vi "SubVI_ResAcc3.vi"() -> (0 "error out":errorcluster caption="에러 출력", 3 "data":waveform(dbl)[](array[waveform]) caption="데이터")   [LabVIEW 2016]
uses:
  <vilib>/DAQmx/read.llb/DAQmx Read.vi
  <vilib>/DAQmx/read.llb/DAQmx Read (Analog 1D Wfm NChan NSamp).vi
  <vilib>/DAQmx/create/channels.llb/DAQmx Create Channel (TEDS-AI-Voltage-Basic).vi
  <vilib>/DAQmx/create/channels.llb/DAQmx Create Channel (AI-Voltage-Basic).vi
  <vilib>/DAQmx/configure/timing.llb/DAQmx Timing (Sample Clock).vi
  <vilib>/DAQmx/configure/trigger.llb/DAQmx Trigger.vi
  <vilib>/DAQmx/configure/trigger.llb/DAQmx Start Trigger (Digital Edge).vi
  <vilib>/DAQmx/miscellaneous.llb/DAQmx Fill In Error Info.vi
panel:
  out "웨이브폼 그래프":waveform(dbl)[](graph)
  out "task out":refnum<k21> caption="태스크 출력"
  in  "error in":errorcluster caption="에러 입력"
  in  "stop (T)":bool=TRUE caption="정지(T)"
  in  "속도":dbl=100000.0
  in  "샘플 개수":i32=2000
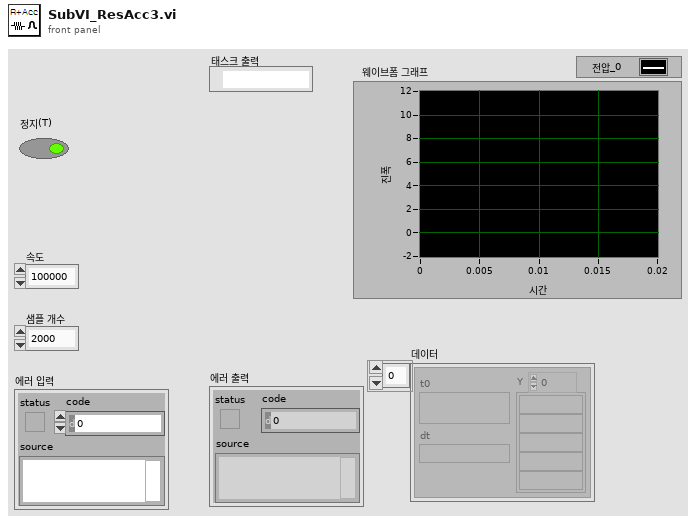
[diagram p1: front panel]
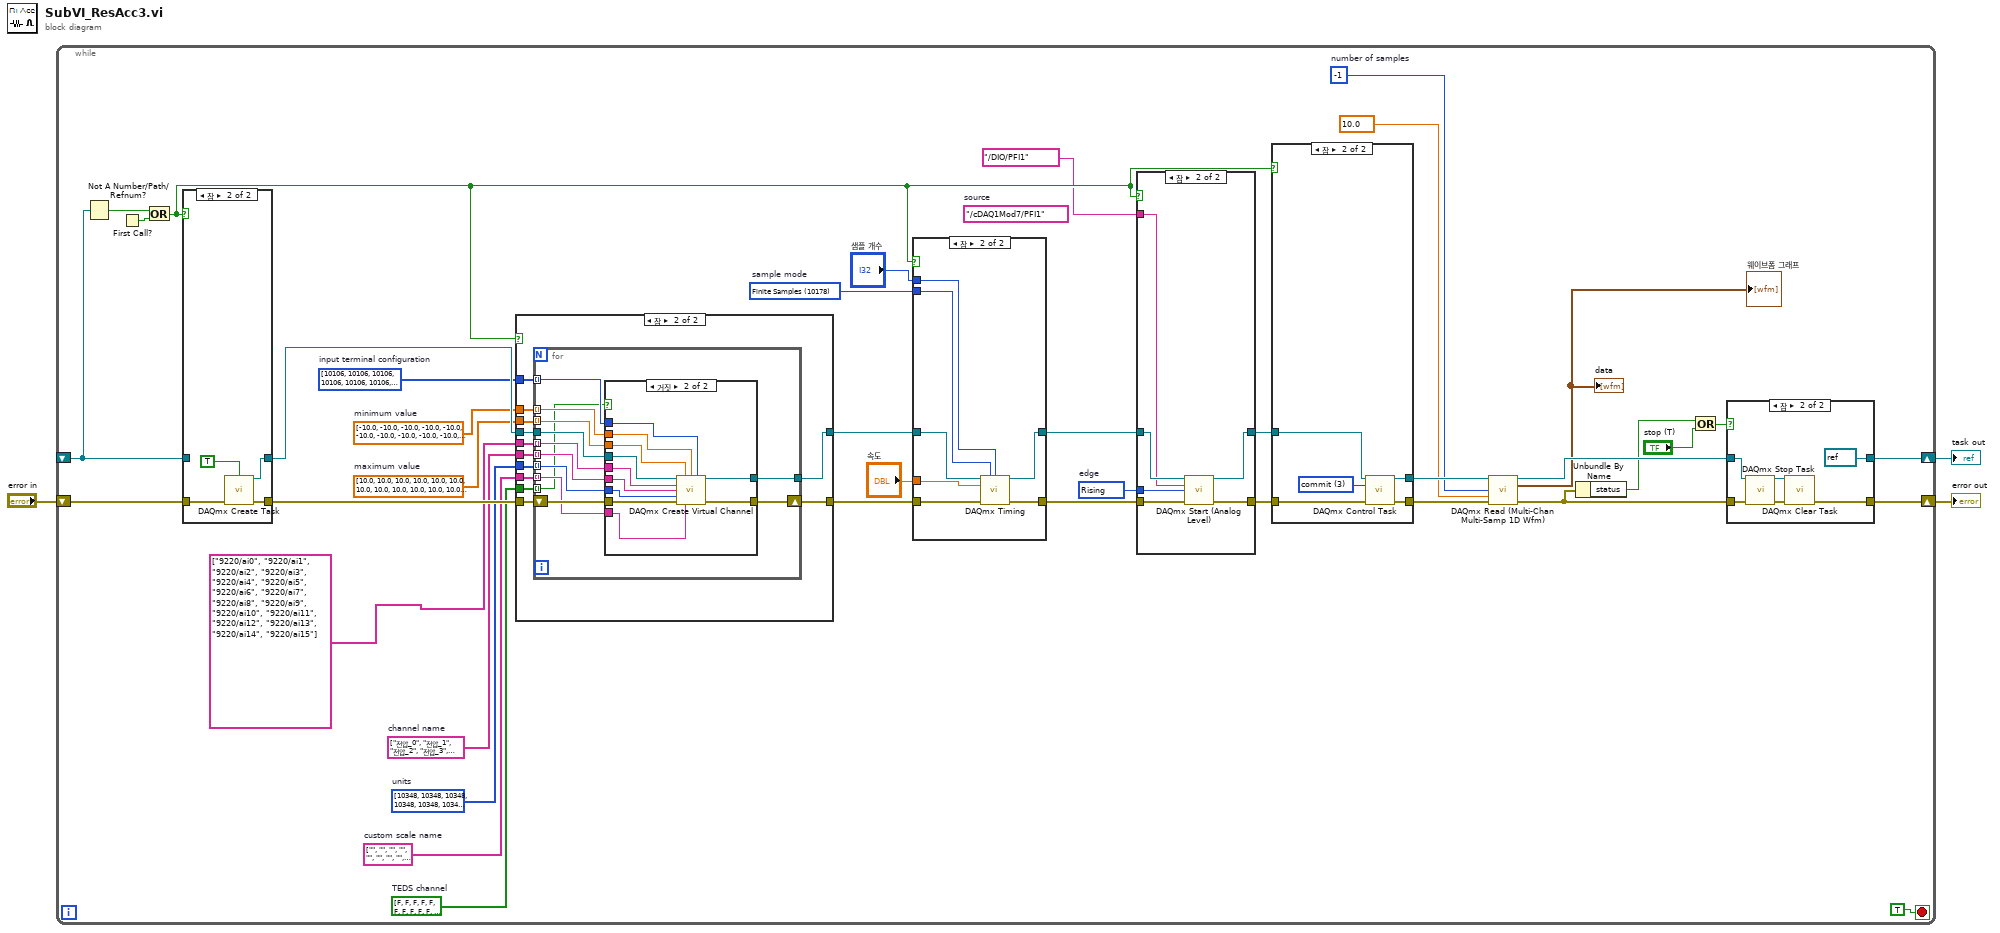
[diagram p0: block diagram]
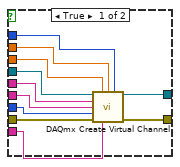
[diagram p7: hidden frame]
diagram:
  n1 = while {
    shift-right: [w12] -> w1
    shift-left: _ -> [w39]
    shift-right: [w10] -> w2
    shift-left: "error in" -> [w40]
    stop <- TRUE stop-if-true
    w14 = -1  # number of samples
    w20 = 10280 items=["Rising"=10280, "Falling"=10171]  # edge
    (unwired) "/cDAQ1Mod7/PFI1"  # source
    w23 = 10178 items=["Finite Samples"=10178, "Continuous Samples"=10123, "Hardware Timed Single Point"=12522]  # sample mode
    w28 = bool[] [FALSE, FALSE, FALSE, FALSE, FALSE, FALSE, FALSE, FALSE, FALSE, FALSE, FALSE, FALSE, FALSE, FALSE, FALSE, FALSE]  # TEDS channel
    w29 = string[] ["", "", "", "", "", "", "", "", "", "", "", "", "", "", "", ""]  # custom scale name
    w30 = i32[] [10348, 10348, 10348, 10348, 10348, 10348, 10348, 10348, 10348, 10348, 10348, 10348, 10348, 10348, 10348, 10348] items=["Volts"=10348, "From TEDS"=12516, "From Custom Scale"=10065]  # units
    w31 = string[] ["전압_0", "전압_1", "전압_2", "전압_3", "전압_4", "전압_5", "전압_6", "전압_7", "전압_8", "전압_9", "전압_10", "전압_11", "전압_12", "전압_13", "전압_14", "전압_15"]  # channel name
    w33 = dbl[] [10.0, 10.0, 10.0, 10.0, 10.0, 10.0, 10.0, 10.0, 10.0, 10.0, 10.0, 10.0, 10.0, 10.0, 10.0, 10.0]  # maximum value
    w34 = dbl[] [-10.0, -10.0, -10.0, -10.0, -10.0, -10.0, -10.0, -10.0, -10.0, -10.0, -10.0, -10.0, -10.0, -10.0, -10.0, -10.0]  # minimum value
    w35 = i32[] [10106, 10106, 10106, 10106, 10106, 10106, 10106, 10106, 10106, 10106, 10106, 10106, 10106, 10106, 10106, 10106] items=["default"=-1, "RSE"=10083, "NRSE"=10078, "Differential"=10106, "Pseudodifferential"=12529]  # input terminal configuration
    n2 = Not A Number/Path/Refnum?(number/path/refnum=w39) -> (NaN/Path/Refnum?=w38:bool)
    n3 = First Call?() -> (First Call?: T/F=w41:bool)
    n4 = Or(x=w38, y=w41) -> (x .or. y?=w19:bool)
    n5 = case "케이스 구조" shown="참" w19 {
      tunnel: [w124 w128] -> w37
      tunnel: w39 -> [w124 _]
      tunnel: [w123 w127] -> w36
      tunnel: w40 -> [w123 w125]
      frame False {
      }
      frame True {
        n6 = call <vilib>:"DAQmx Create Task.vi"("auto cleanup"=TRUE, "error in"=w125) -> ("task out"=w128:refnum<k21>, "error out"=w127:errorcluster)  [unwired: 12 in]
      }
    }
    n7 = case "케이스 구조" shown="참" w19 {
      tunnel: [w76 w86] -> w27
      tunnel: w37 -> [w76 w88]
      tunnel: [w75 w85] -> w26
      tunnel: w36 -> [w75 w87]
      tunnel: w35 -> [_ w84]
      tunnel: w34 -> [_ w83]
      tunnel: w33 -> [_ w82]
      tunnel: tag[] ["9220/ai0", "9220/ai1", "9220/ai2", "9220/ai3", "9220/ai4", "9220/ai5", "9220/ai6", "9220/ai7", "9220/ai8", "9220/ai9", "9220/ai10", "9220/ai11", "9220/ai12", "9220/ai13", "9220/ai14", "9220/ai15"] -> [_ w81]
      tunnel: w31 -> [_ w80]
      tunnel: w30 -> [_ w79]
      tunnel: w29 -> [_ w78]
      tunnel: w28 -> [_ w77]
      frame False {
      }
      frame True {
        n8 = for "For 루프" {
          tunnel: w88 -> [w100]
          tunnel: [w98] -> w86
          tunnel: w84 -> [w96] mode=indexing
          tunnel: w83 -> [w95] mode=indexing
          tunnel: w82 -> [w94] mode=indexing
          tunnel: w81 -> [w93] mode=indexing
          tunnel: w80 -> [w92] mode=indexing
          tunnel: w79 -> [w91] mode=indexing
          tunnel: w78 -> [w90] mode=indexing
          shift-right: [w97] -> w85
          shift-left: w87 -> [w99]
          tunnel: w77 -> [w89] mode=indexing
          n9 = case "케이스 구조" shown="거짓" w89 {
            tunnel: w100 -> [w111 w122]
            tunnel: w99 -> [w110 w121]
            tunnel: [w109 w120] -> w98
            tunnel: [w108 w119] -> w97
            tunnel: w96 -> [w107 w118]
            tunnel: w95 -> [w106 w117]
            tunnel: w94 -> [w105 w116]
            tunnel: w93 -> [w104 w115]
            tunnel: w92 -> [w103 w114]
            tunnel: w91 -> [w102 w113]
            tunnel: w90 -> [w101 w112]
            frame True {
              n10 = call-poly <vilib>:"DAQmx Create Virtual Channel.vi"("task in"=w111, "maximum value"=w105, "minimum value"=w106, "input terminal configuration"=w107, "physical channels"=w104, "name to assign"=w103, "units"=w102, "error in"=w110, "custom scale name"=w101) -> ("task out"=w109:refnum<k21>, "error out"=w108:errorcluster)  [unwired: 5 in]
            }
            frame False {
              n11 = call-poly <vilib>:"DAQmx Create Virtual Channel.vi"("task in"=w122, "maximum value"=w116, "minimum value"=w117, "input terminal configuration"=w118, "physical channels"=w115, "name to assign"=w114, "units"=w113, "error in"=w121, "custom scale name"=w112) -> ("task out"=w120:refnum<k21>, "error out"=w119:errorcluster)  [unwired: 5 in]
            }
          }
        }
      }
    }
    n12 = case "케이스 구조" shown="참" w19 {
      tunnel: [w67 w69] -> w22
      tunnel: w27 -> [w67 w72]
      tunnel: [w66 w68] -> w21
      tunnel: w26 -> [w66 w70]
      tunnel: "샘플 개수" -> [_ w74]
      tunnel: w23 -> [_ w73]
      tunnel: "속도" -> [_ w71]
      frame False {
      }
      frame True {
        n13 = call-poly <vilib>:"DAQmx Timing.vi"("task/channels in"=w72, "sample mode"=w73, "samples per channel"=w74, "rate"=w71, "error in"=w70) -> ("task out"=w69:refnum<k21>, "error out"=w68:errorcluster)  [unwired: 9 in]
      }
    }
    n14 = case "케이스 구조" shown="참" w19 {
      tunnel: [w59 w63] -> w18
      tunnel: w22 -> [w59 w65]
      tunnel: [w58 w62] -> w17
      tunnel: w21 -> [w58 w64]
      tunnel: tag "/DIO/PFI1" ("source") -> [_ w61]
      tunnel: w20 -> [_ w60]
      frame False {
      }
      frame True {
        n15 = call-poly "DAQmx Start (Analog Level).vi"("task/channels in"=w65, "source"=w61, "edge"=w60, "error in"=w64) -> ("task out"=w63:refnum<k21>, "error out"=w62:errorcluster)  [unwired: 10 in]
      }
    }
    n16 = case "케이스 구조" shown="참" w19 {
      tunnel: [w52 w56] -> w16
      tunnel: w18 -> [w52 w57]
      tunnel: [w51 w54] -> w15
      tunnel: w17 -> [w51 w55]
      frame False {
      }
      frame True {
        w53 = 3 items=["verify"=2, "reserve"=4, "commit"=3, "unreserve"=5, "abort"=6] ("action")
        n17 = call <vilib>:"DAQmx Control Task.vi"("task/channels in"=w57, "action"=w53, "error in"=w55) -> ("task out"=w56:refnum<k21>, "error out"=w54:errorcluster)  [unwired: 11 in]
      }
    }
    n18 = call-poly "DAQmx Read (Multi-Chan Multi-Samp 1D Wfm).vi"("task/channels in"=w16, "number of samples per channel"=w14, "timeout"=10.0 ("timeout (s)"), "error in"=w15) -> ("task out"=w11:refnum<k21>, "data"=→"data" →"웨이브폼 그래프":waveform(dbl)[], "error out"=w9:errorcluster)  [unwired: 9 in]
    n19 = Unbundle By Name(w9) -> ("status"=w8:bool)
    n20 = Or(x=w8, y="stop (T)") -> (x .or. y?=w6:bool)
    n21 = case "케이스 구조" shown="참" w6 {
      tunnel: [w44 refnum<k21> refnum ("task in")] -> w12
      tunnel: w11 -> [w44 w50]
      tunnel: [w43 w47] -> w10
      tunnel: w9 -> [w43 w49]
      frame False {
      }
      frame True {
        n22 = call <vilib>:"DAQmx Stop Task.vi"("task/channels in"=w50, "error in"=w49) -> ("task out"=w46:refnum<k21>, "error out"=w48:errorcluster)  [unwired: 12 in]
        n23 = call <vilib>:"DAQmx Clear Task.vi"("task in"=w46, "error in"=w48) -> ("error out"=w47:errorcluster)  [unwired: 13 in]
      }
    }
  }
  "error out" <- w2
  "task out" <- w1
